vi "3.0-State Update.vi"() -> (0 "End Program":bool)   [LabVIEW 2010]
uses:
  <vilib>/Platform/TimedLoop/XDataNode/XDataNode.xnode
  <vilib>/Platform/TimedLoop/XDataNode/timing_clust.ctl
  <vilib>/Platform/TimedLoop/XDataNode/nitl_modes.ctl
  <vilib>/Platform/TimedLoop/XDataNode/wakeup.ctl
  3.0 List of Loops.ctl
  4-High Neurons/4.0-Midbrain State.ctl
  2-Low Neurons/2.0-Hindbrain Startup State.ctl
  <vilib>/rvi/interface/nirviReadWriteControl/nirviReadWriteControl.xnode
  FPGA Bitfiles/1Hindbrain.lvbitx
  1-Hindbrain.vi
  <vilib>/rvi/interface/common/niFpgaNodeNameForErrorReporting.ctl
  <vilib>/rvi/errors/niLvFpgaWhatHappensToTopLevelVI.ctl
  3.0-Global.vi
  <vilib>/Utility/error.llb/Error Cluster From Error Code.vi
  <vilib>/rvi/errors/niLvFpgaAdjustHostInterfaceError.vi
  NiFpgaLv.dll
  <vilib>/Platform/TimedLoop/XDataNode/XDNodeRunTimeDep.lvlib
panel:
  out "Pointer to FPGA":u32
  out "Has Refrence":bool
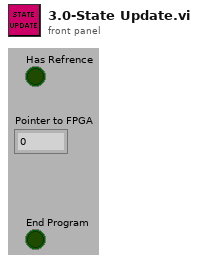
[diagram p1: front panel]
types:
  T1 = typedef "XDNodeRunTimeDep.lvlib/timing_clust.ctl" = cluster{"Expected End [f-1]":u64, "Actual End [f-1]":u64, "Finished Late? [f-1]":bool, "Expected End [i-1]":u64, "Actual End [i-1]":u64, "Finished Late? [i-1]":bool, "Expected Start [i]":u64, "Actual Start [i]":u64, "Expected Start [f]":u64, "Actual Start [f]":u64, "Source Name":string, "Structure Name":string, "Period":i64, "Deadline":i64, "Offset":i64, "Start":i64, "Priority":i32, "Timeout":i32, "Mode":T2, "Wakeup Reason":T3, "Error":errorcluster, "Source Type":string, "Secondary Source Type":string, "Global End Time":u64, "Global Start Time":u64, "Frame Duration":u64, "Iteration Duration":u64, "Assigned CPU":i32, "I/O Scan Engine Mode":u32}
  T2 = typedef "XDNodeRunTimeDep.lvlib/nitl_modes.ctl" = enum32{"No Change", "Process missed periods, maintain original phase", "Discard missed periods, maintain original phase", "Process missed periods, ignore original phase", "Discard missed periods, ignore original phase"}
  T3 = typedef "XDNodeRunTimeDep.lvlib/wakeup.ctl" = enum32{"Normal", "Aborted", "Asynchronous wakeup", "Timing source error", "Timed loop error", "Timeout"}
  T4 = typedef "3.0 List of Loops.ctl" = enum16{"3.0 State Update", "3.0 GUI", "3.1 Act", "3.1 4.7.1 Act UDP", "3.1 Joystick", "3.2 Where", "3.2.0 Kalman Filter", "3.2 4.7.2 Where UDP", "3.3 What", "3.3 4.7.3 What UDP", "3.4 How", "3.4 4.7.4 How UDP", "3.5 Limbic", "3.8 TCP", "3.6 Cerebellum", "3.8 TCP Act", "3.11 Shallow Map", "3.1.17 Decider"}
  T5 = typedef "4.0-Midbrain State.ctl" = enum16{"Startup", "Waiting to Run", "Running-OlinOval", "Running-ChannelFollow", "Running-WallFollow", "Running-OpenTransit", "Running-Joystick Training", "Shutdown", "Restart"}
  T6 = typedef "2.0-Hindbrain Startup State.ctl" = enum8{"Waiting to Run", "Running", "Restart", "Shutdown", "Off"}
  T7 = typedef "niFpgaNodeNameForErrorReporting.ctl" = enum16{"Open FPGA VI Reference", "Read/Write Control", "Invoke Method: Abort", "Invoke Method: Acknowledge IRQ", "Invoke Method: Download", "Invoke Method: FIFO.Configure", "Invoke Method: FIFO.Read", "Invoke Method: FIFO.Start", "Invoke Method: FIFO.Stop", "Invoke Method: FIFO.Write", "Invoke Method: Reset", "Invoke Method: Run", "Invoke Method: Wait on IRQ", "Close FPGA VI Reference"}
  T8 = typedef "niLvFpgaWhatHappensToTopLevelVI.ctl" = enum16{"top level VI scripted behind XNode", "top level VI inlined behind XNode"}
  T9 = typedef "4.1-Act Control Typedef.ctl" = cluster{"E-Stop":bool, "Restart":bool, "Extended Joystick":bool, "Begin":bool, "Time":i32, "Shutdown":bool, "Saitek Controler":T10, "Joystick Valid":bool}
  T10 = typedef "6.1-UDP Saitek.ctl" = cluster{"Stop":bool, "Setpoint":bool, "Run":bool, "Restart":bool, "Shutdown":bool, "Joystick\nMode 1":bool, "Joystick\nMode 2":bool, "Joystick \nMode 3":bool, "Joystick Mode 4":bool, "10":bool, "11":bool, "Pitch":sgl, "Roll":sgl, "Yaw":sgl, "Left":sgl, "Right":sgl}
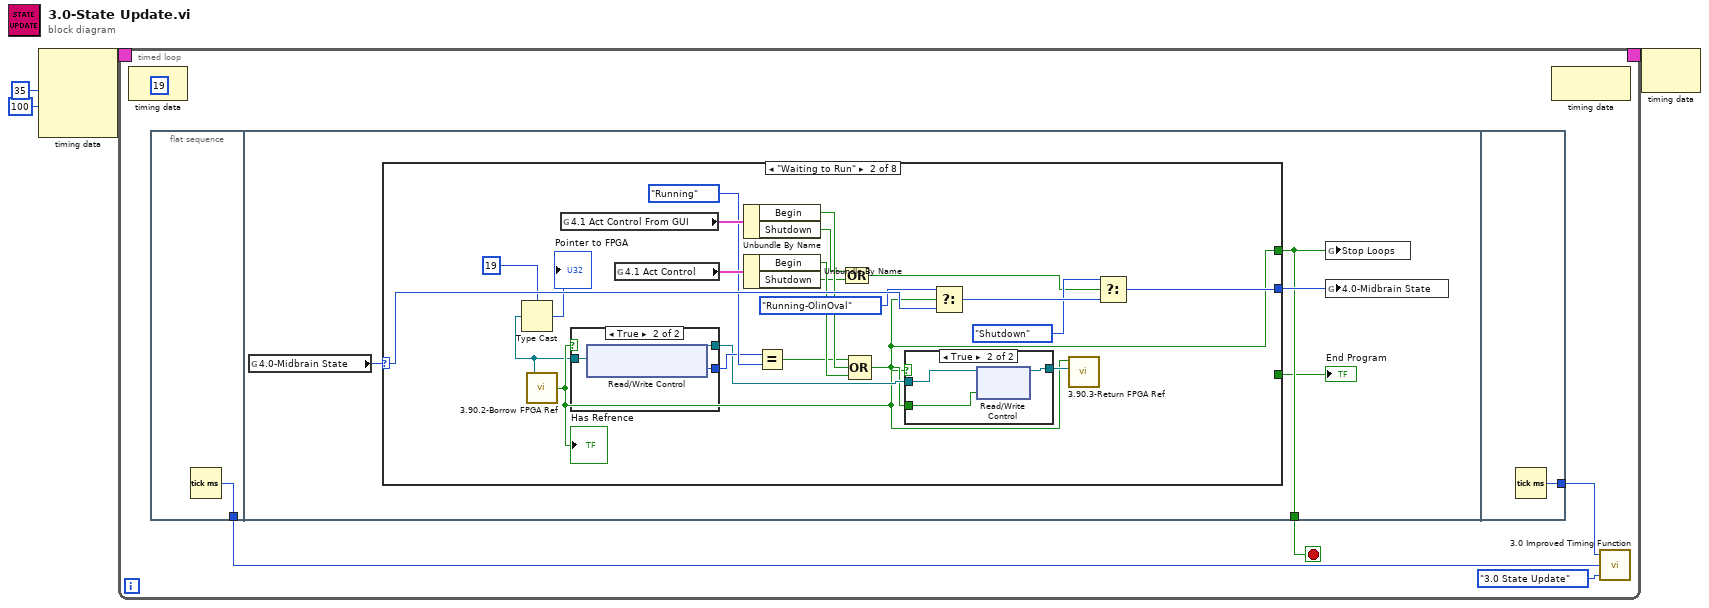
[diagram p0: block diagram]
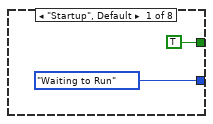
[diagram p2: hidden frame]
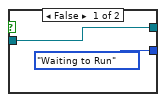
[diagram p4: hidden frame]
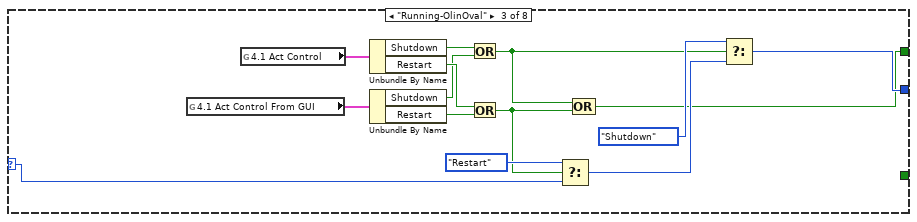
[diagram p5: hidden frame]
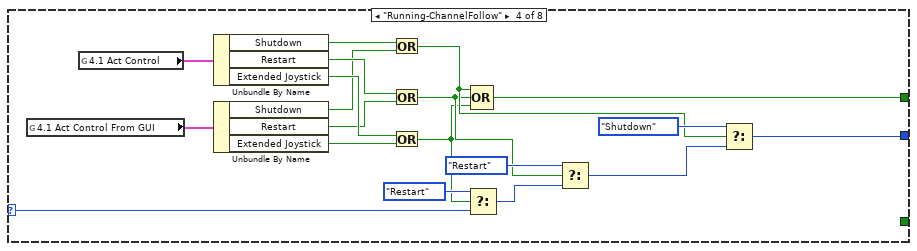
[diagram p6: hidden frame]
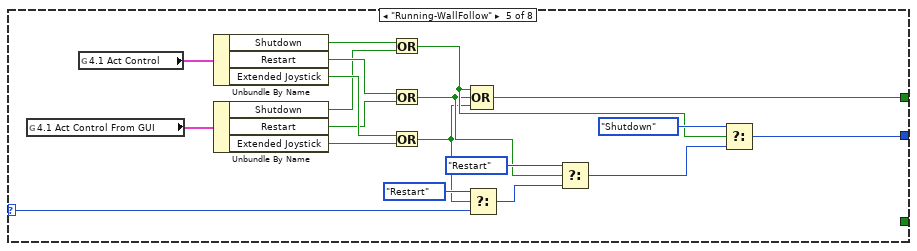
[diagram p7: hidden frame]
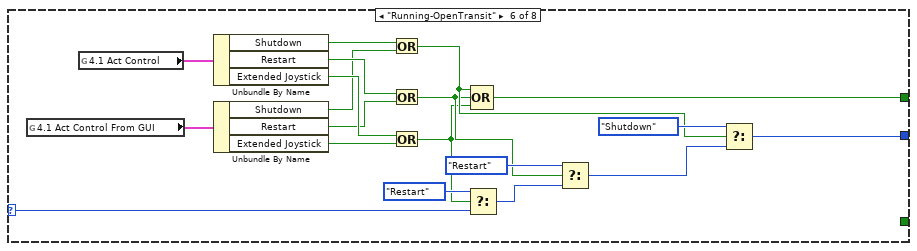
[diagram p8: hidden frame]
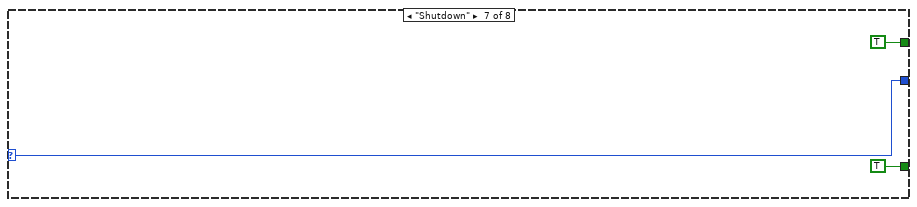
[diagram p9: hidden frame]
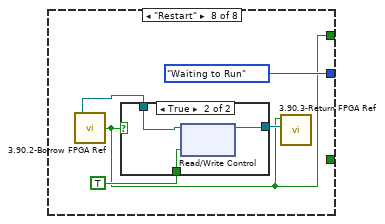
[diagram p10: hidden frame]
diagram:
  n1 = node-c288(i64 35 ("Period"), 100 ("Priority")) -> (w4:T1)  [unwired: 2 in]
  n2 = timed-loop {
    timing: w4 -> [_]
    timing-out: [_] -> w3
    stop <- w8 stop-if-true
    (unwired) u32 19 ("millisecond multiple")
    n3 = node-c288() -> ()  [unwired: 1 in, 1 out]
    n4 = flat-sequence {
      tunnel: [w11] -> w6
      tunnel: [w13] -> w8
      tunnel: [w247] -> w7
      frame #0 {
        n5 = Tick Count (ms)() -> (millisecond timer value=w11:u32)
      }
      frame #1 {
        n6 = global read "3.0-Global.vi" "4.0-Midbrain State"() -> (w15:T5)
        n7 = case shown="\"Waiting to Run\"" w15 {
          selector: w15 -> [_ w38 w126 w157 w176 w195 w199 _]
          tunnel: [4.0-Midbrain_State."Waiting to Run" ("4.0-Midbrain State 3") w28 w135 w151 w170 w189 w199 4.0-Midbrain_State."Waiting to Run" ("4.0-Midbrain State")] -> w14
          tunnel: [TRUE w22 w132 w147 w166 w185 TRUE ("Begin") w200] -> w13
          tunnel: [_ _ _ _ _ _ TRUE ("Stop Loops") _] -> w12
          frame "Startup", Default {
          }
          frame "Waiting to Run" {
            n8 = call "3.90.2-Borrow FPGA Ref.vi"() -> ("Has Refrence"=w21:bool, "Ref Out"=w19:refnum<k20>)
            "Has Refrence" <- w21
            n9 = Type Cast(type=u32 19 ("millisecond multiple"), x=w19) -> (*(type *) &x=→"Pointer to FPGA":u32)
            n10 = global read "3.0-Global.vi" "4.1 Act Control From GUI"() -> (w36:T9)
            n11 = case shown="True" w21 {
              tunnel: w19 -> [w83 w86]
              tunnel: [w83 w85] -> w24
              tunnel: [2.0-Hindbrain_Startup_State."Waiting to Run" ("1.0-Hindbrain State") w84] -> w32
              frame False {
              }
              frame True {
                n12 = xnode "Read/Write Control"("FPGA VI Reference In"=w86) -> ("FPGA VI Reference Out"=w85:refnum<k20>, "1.0-Hindbrain State"=w84:T6)  [unwired: 1 in, 1 out]
              }
            }
            n13 = global read "3.0-Global.vi" "4.1 Act Control"() -> (w39:T9)
            n14 = Unbundle By Name(w36) -> ("Begin"=w35:bool, "Shutdown"=w26:bool)
            n15 = Unbundle By Name(w39) -> ("Begin"=w34:bool, "Shutdown"=w27:bool)
            n16 = Equal?(x=w32, y=2.0-Hindbrain_Startup_State."Running") -> (x = y?=w31:bool)
            n17 = Compound Arithmetic op=OR(w26, w27) -> (w25:bool)
            n18 = Compound Arithmetic op=OR(w31, w35, w34) -> (w22:bool)
            n19 = case shown="True" w21 {
              tunnel: w24 -> [w40 w43]
              tunnel: [w40 w42] -> w23
              tunnel: w22 -> [_ w41]
              frame False {
              }
              frame True {
                n20 = xnode "Read/Write Control"("FPGA VI Reference In"=w43, "Begin"=w41) -> ("FPGA VI Reference Out"=w42:refnum<k20>)  [unwired: 1 in, 1 out]
              }
            }
            n21 = Select(t=4.0-Midbrain_State."Running-OlinOval", s=w22, f=w38) -> (s? t:f=w30:T5)
            n22 = call "3.90.3-Return FPGA Ref.vi"("element"=w23, "Has Refrence"=w21) -> ()  [unwired: 3 in]
            n23 = Select(t=4.0-Midbrain_State."Shutdown", s=w25, f=w30) -> (s? t:f=w28:T5)
          }
          frame "Running-OlinOval" {
            n24 = global read "3.0-Global.vi" "4.1 Act Control From GUI"() -> (w131:T9)
            n25 = global read "3.0-Global.vi" "4.1 Act Control"() -> (w139:T9)
            n26 = Unbundle By Name(w139) -> ("Shutdown"=w134:bool, "Restart"=w133:bool)
            n27 = Unbundle By Name(w131) -> ("Shutdown"=w128:bool, "Restart"=w127:bool)
            n28 = Or(x=w134, y=w128) -> (x .or. y?=w130:bool)
            n29 = Or(x=w133, y=w127) -> (x .or. y?=w129:bool)
            n30 = Select(t=4.0-Midbrain_State."Restart", s=w129, f=w126) -> (s? t:f=w138:T5)
            n31 = Compound Arithmetic op=OR(w130, w129) -> (w132:bool)
            n32 = Select(t=4.0-Midbrain_State."Shutdown", s=w130, f=w138) -> (s? t:f=w135:T5)
          }
          frame "Running-ChannelFollow" {
            n33 = global read "3.0-Global.vi" "4.1 Act Control From GUI"() -> (w146:T9)
            n34 = global read "3.0-Global.vi" "4.1 Act Control"() -> (w158:T9)
            n35 = Unbundle By Name(w158) -> ("Shutdown"=w150:bool, "Restart"=w149:bool, "Extended Joystick"=w148:bool)
            n36 = Unbundle By Name(w146) -> ("Shutdown"=w142:bool, "Restart"=w141:bool, "Extended Joystick"=w140:bool)
            n37 = Or(x=w150, y=w142) -> (x .or. y?=w145:bool)
            n38 = Or(x=w149, y=w141) -> (x .or. y?=w144:bool)
            n39 = Or(x=w148, y=w140) -> (x .or. y?=w143:bool)
            n40 = Select(t=4.0-Midbrain_State."Restart", s=w143, f=w157) -> (s? t:f=w156:T5)
            n41 = Compound Arithmetic op=OR(w145, w144, w143) -> (w147:bool)
            n42 = Select(t=4.0-Midbrain_State."Restart", s=w144, f=w156) -> (s? t:f=w155:T5)
            n43 = Select(t=4.0-Midbrain_State."Shutdown", s=w145, f=w155) -> (s? t:f=w151:T5)
          }
          frame "Running-WallFollow" {
            n44 = global read "3.0-Global.vi" "4.1 Act Control From GUI"() -> (w165:T9)
            n45 = global read "3.0-Global.vi" "4.1 Act Control"() -> (w177:T9)
            n46 = Unbundle By Name(w177) -> ("Shutdown"=w169:bool, "Restart"=w168:bool, "Extended Joystick"=w167:bool)
            n47 = Unbundle By Name(w165) -> ("Shutdown"=w161:bool, "Restart"=w160:bool, "Extended Joystick"=w159:bool)
            n48 = Or(x=w169, y=w161) -> (x .or. y?=w164:bool)
            n49 = Or(x=w168, y=w160) -> (x .or. y?=w163:bool)
            n50 = Or(x=w167, y=w159) -> (x .or. y?=w162:bool)
            n51 = Select(t=4.0-Midbrain_State."Restart", s=w162, f=w176) -> (s? t:f=w175:T5)
            n52 = Compound Arithmetic op=OR(w164, w163, w162) -> (w166:bool)
            n53 = Select(t=4.0-Midbrain_State."Restart", s=w163, f=w175) -> (s? t:f=w174:T5)
            n54 = Select(t=4.0-Midbrain_State."Shutdown", s=w164, f=w174) -> (s? t:f=w170:T5)
          }
          frame "Running-OpenTransit" {
            n55 = global read "3.0-Global.vi" "4.1 Act Control From GUI"() -> (w184:T9)
            n56 = global read "3.0-Global.vi" "4.1 Act Control"() -> (w196:T9)
            n57 = Unbundle By Name(w196) -> ("Shutdown"=w188:bool, "Restart"=w187:bool, "Extended Joystick"=w186:bool)
            n58 = Unbundle By Name(w184) -> ("Shutdown"=w180:bool, "Restart"=w179:bool, "Extended Joystick"=w178:bool)
            n59 = Or(x=w188, y=w180) -> (x .or. y?=w183:bool)
            n60 = Or(x=w187, y=w179) -> (x .or. y?=w182:bool)
            n61 = Or(x=w186, y=w178) -> (x .or. y?=w181:bool)
            n62 = Select(t=4.0-Midbrain_State."Restart", s=w181, f=w195) -> (s? t:f=w194:T5)
            n63 = Compound Arithmetic op=OR(w183, w182, w181) -> (w185:bool)
            n64 = Select(t=4.0-Midbrain_State."Restart", s=w182, f=w194) -> (s? t:f=w193:T5)
            n65 = Select(t=4.0-Midbrain_State."Shutdown", s=w183, f=w193) -> (s? t:f=w189:T5)
          }
          frame "Shutdown" {
          }
          frame "Restart" {
            n66 = call "3.90.2-Borrow FPGA Ref.vi"() -> ("Has Refrence"=w200:bool, "Ref Out"=w201:refnum<k20>)
            n67 = case shown="True" w200 {
              tunnel: [w205 w207] -> w203
              tunnel: TRUE ("Begin") -> [_ w208]
              tunnel: w201 -> [w205 w206]
              frame False {
              }
              frame True {
                n68 = xnode "Read/Write Control"("FPGA VI Reference In"=w206, "Restart"=w208) -> ("FPGA VI Reference Out"=w207:refnum<k20>)  [unwired: 1 in, 1 out]
              }
            }
            n69 = call "3.90.3-Return FPGA Ref.vi"("element"=w203, "Has Refrence"=w200) -> ()  [unwired: 3 in]
          }
        }
        "End Program" <- w12
        n70 = global write "3.0-Global.vi" "Stop Loops"(w13) -> ()
        n71 = global write "3.0-Global.vi" "4.0-Midbrain State"(w14) -> ()
      }
      frame #2 {
        n72 = Tick Count (ms)() -> (millisecond timer value=w247:u32)
      }
    }
    n73 = node-c288() -> ()  [unwired: 1 in, 1 out]
    n74 = call "3.0 Improved Timing Function.vi"("Loop"=3.0_List_of_Loops."3.0 State Update", "Start"=w6, "End"=w7) -> ()  [unwired: 1 in]
  }
  n75 = node-c288(w3) -> ()  [unwired: 1 out]
